vi "CANOpen_SDO List RW.vi"(8 "error in (no error)":errorcluster, 11 "SDO Asynch in":T1 {"HW Dyn Read"."Resp Chan."."Chan Refs" format="%.0x"; "HW Dyn Read"."Req Chan."."Chan Refs" format="%.0x"; "HW Dyn Write"."Resp Chan."."Chan Refs" format="%.0x"; "HW Dyn Write"."Req Chan."."Chan Refs" format="%.0x"; "List SDO"."Resp Chan."."Chan Refs" format="%.0x"; "List SDO"."Req Chan."."Chan Refs" format="%.0x"}) -> (0 "error out":errorcluster, 3 "SDO Asynch out":T1 {"HW Dyn Read"."Resp Chan."."Chan Refs" format="%.0x"; "HW Dyn Read"."Req Chan."."Chan Refs" format="%.0x"; "HW Dyn Write"."Resp Chan."."Chan Refs" format="%.0x"; "HW Dyn Write"."Req Chan."."Chan Refs" format="%.0x"; "List SDO"."Resp Chan."."Chan Refs" format="%.0x"; "List SDO"."Req Chan."."Chan Refs" format="%.0x"})   [LabVIEW 2021, in "CANOpen Addon Engine.lvlib"]
uses:
  CANOpen Addon Engine.lvlib
  CANOpen_VS SDOs Data Refs.ctl
  <vilib>/NI VeriStand/Custom Device API/Data Reference.ctl
  Async VIs/CANOpen_Main/SubVIs/CanOpen_SDO Dynamic queue.ctl
  Shared/CANOpen_SDO queue W data.ctl
  Shared/CANOpen_SDO queue mode.ctl
  Shared/CANOpen_PDO Data Type in queue.ctl
  <vilib>/NI VeriStand/Custom Device API/Global Data Refs.vi
  <vilib>/NI VeriStand/Custom Device API/Custom Device API.lvlib
  Debug/SubVIs/Global debug.vi
  <vilib>/NI VeriStand/Custom Device Tools/Custom Device Utility Library/Custom Device Utility Library.lvlib
  Shared/CANOpen Addon Shared.lvlib
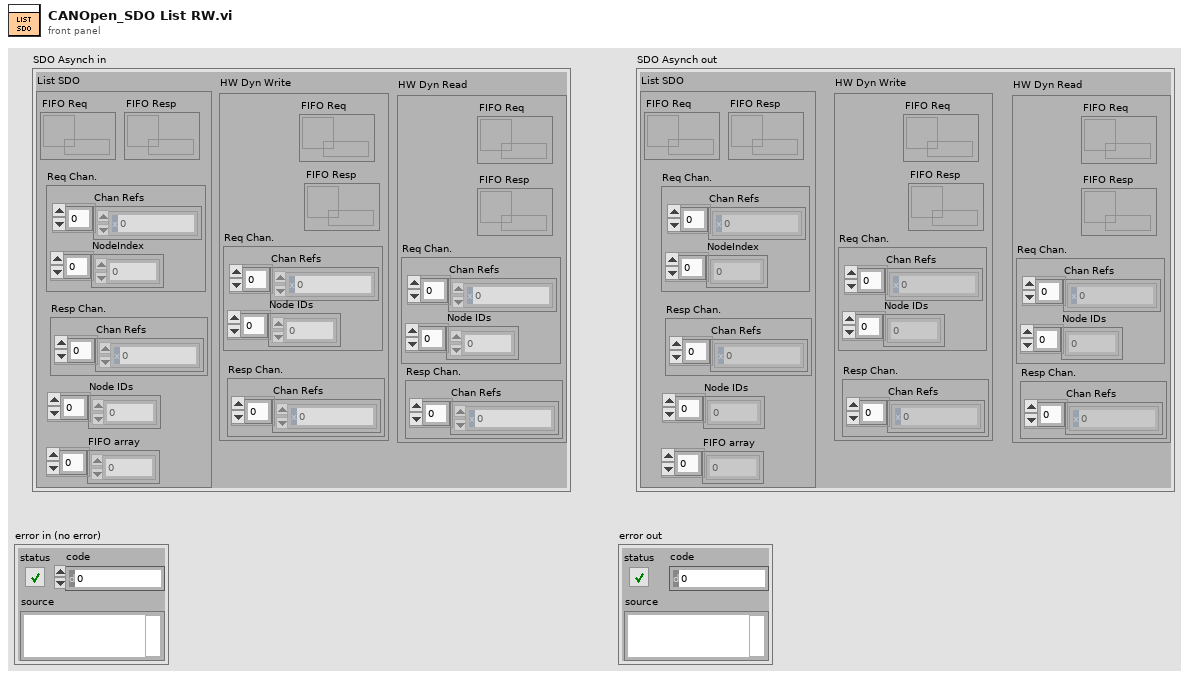
[diagram p1: front panel]
types:
  T1 = typedef "CANOpen Addon Engine.lvlib/CANOpen_VS SDOs Data Refs.ctl" = cluster{"List SDO":cluster{"FIFO Req":refnum<k33>, "Req Chan.":cluster{"Chan Refs":T2[], "NodeIndex":dbl[]}, "FIFO Resp":refnum<k33>, "Resp Chan.":cluster{"Chan Refs":T2[]}, "Node IDs":u8[], "FIFO array":dbl[]}, "HW Dyn Write":cluster{"FIFO Req":refnum<k33>, "FIFO Resp":refnum<k33>, "Req Chan.":cluster{"Chan Refs":T2[], "Node IDs":u8[]}, "Resp Chan.":cluster{"Chan Refs":T2[]}}, "HW Dyn Read":cluster{"FIFO Req":refnum<k33>, "FIFO Resp":refnum<k33>, "Req Chan.":cluster{"Chan Refs":T2[], "Node IDs":u8[]}, "Resp Chan.":cluster{"Chan Refs":T2[]}}}
  T2 = typedef "Custom Device API.lvlib/Data Reference.ctl" = i32
  T3 = typedef "CANOpen Addon Engine.lvlib/CanOpen_SDO Dynamic queue.ctl" = cluster{"Node ID":u8, "Data":T4}
  T4 = typedef "CANOpen Addon Shared.lvlib/CANOpen_SDO queue W data.ctl" = cluster{"Object Index":u16, "Object Sub-Index (0)":u8, "Mode":T5, "Data Type":T6, "Value":dbl, "Status code":dbl, "Byte Order":enum16{"big-endian, network order", "little-endian"}}
  T5 = typedef "CANOpen Addon Shared.lvlib/CANOpen_SDO queue mode.ctl" = enum16{"WRITE write", "WRITE response", "READ write", "READ response"}
  T6 = typedef "CANOpen Addon Shared.lvlib/CANOpen_PDO Data Type in queue.ctl" = enum16{"U8", "U16", "U32", "I8", "I16", "I32", "Single", "Double"}
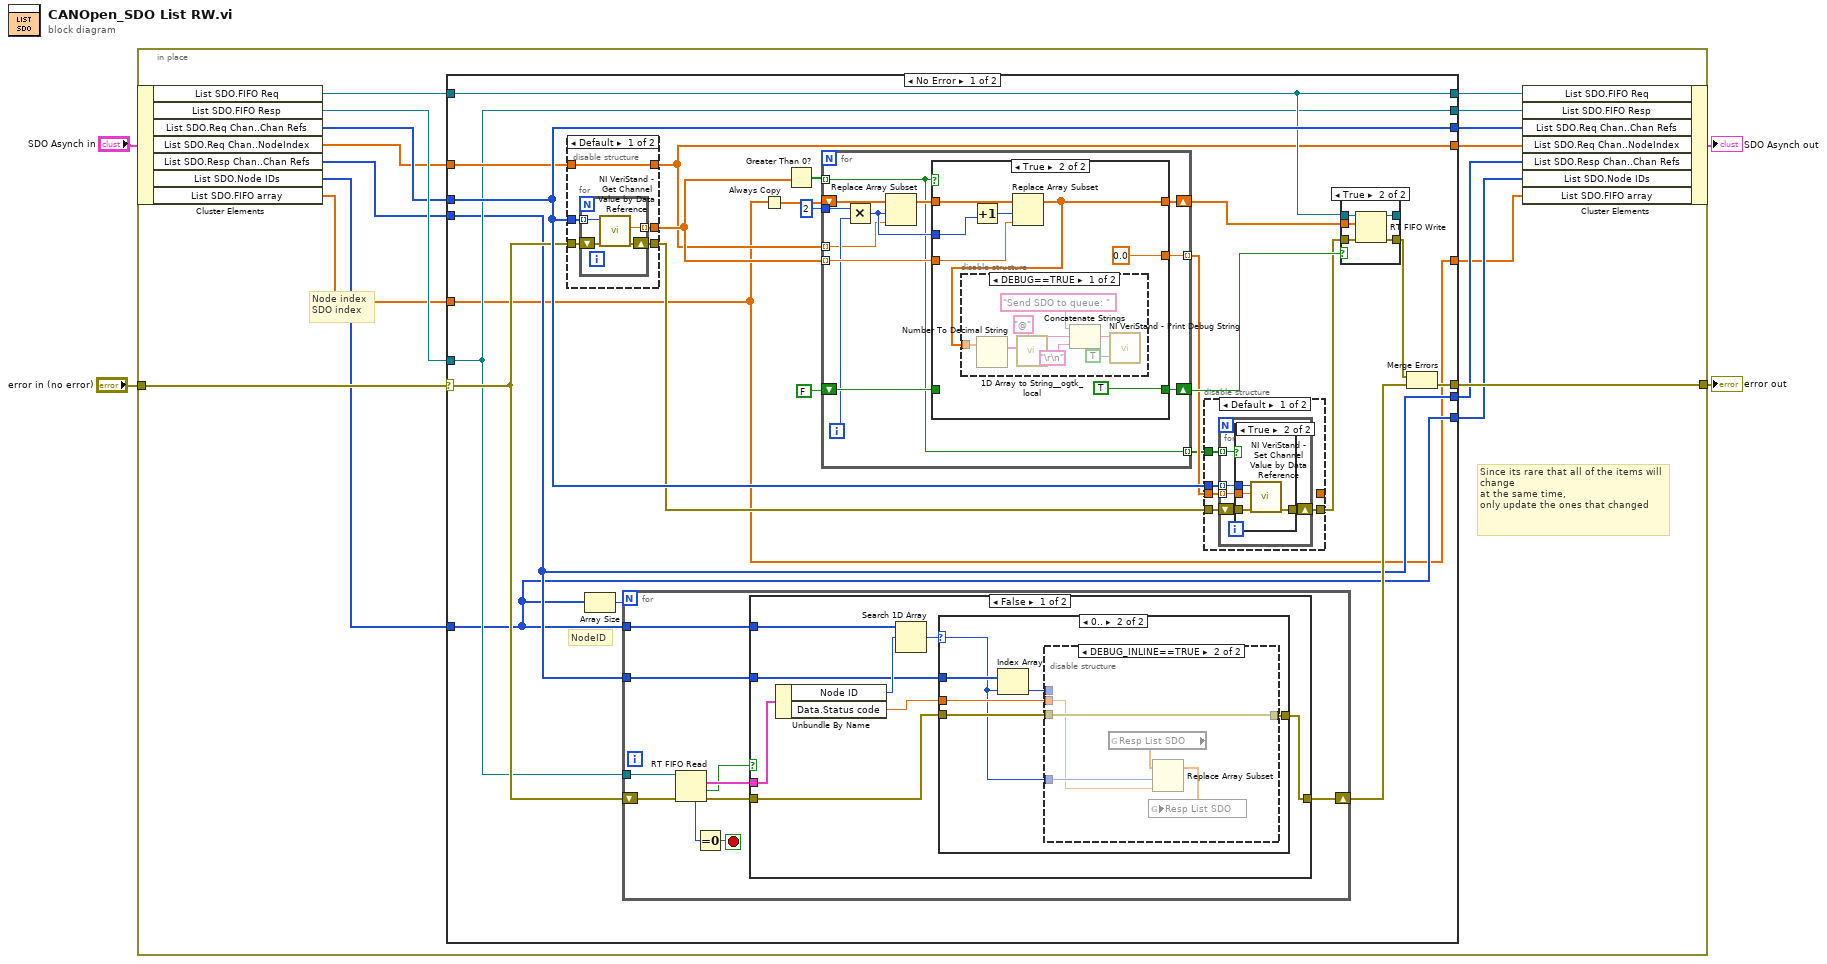
[diagram p0: block diagram]
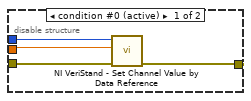
[diagram p3: hidden frame]
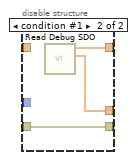
[diagram p5: hidden frame]
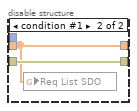
[diagram p7: hidden frame]
diagram:
  n1 = in-place {
    in-place-border: "error in (no error)" -> [w15]
    in-place-border: [w14] -> w1
    # "Since its rare that all of the items will change \nat the same time,\nonly update the ones that changed"
    # "Node index\nSDO index"
    n2 = in-place-cluster #1("SDO Asynch in") -> ("List SDO.FIFO Req"=w16:refnum<k33>, "List SDO.FIFO Resp"=w20:refnum<k33>, "List SDO.Req Chan..Chan Refs"=w18:T2[], "List SDO.Req Chan..NodeIndex"=w13:dbl[], "List SDO.Resp Chan..Chan Refs"=w9:T2[], "List SDO.Node IDs"=w7:u8[], "List SDO.FIFO array"=w6:dbl[])
    n3 = case shown="No Error" w15 {
      selector: w15 -> [w28 w149]
      tunnel: [w32 w149] -> w14
      tunnel: w20 -> [w27 w153]
      tunnel: [w27 w153] -> w19
      tunnel: w18 -> [w44 w152]
      tunnel: w13 -> [w29 w151]
      tunnel: [w44 w152] -> w17
      tunnel: [w25 w151] -> w12
      tunnel: w16 -> [w43 w150]
      tunnel: w9 -> [w26 w148]
      tunnel: [w43 w150] -> w11
      tunnel: [w26 w148] -> w10
      tunnel: w7 -> [w24 w147]
      tunnel: [w24 w147] -> w8
      tunnel: w6 -> [w21 w146]
      tunnel: [w21 w146] -> w5
      frame No Error {
        # "NodeID"
        n4 = disable-structure shown="Default" {
          disable-tunnel: w44 -> [w84 _]
          disable-tunnel: w28 -> [w83 w89]
          disable-tunnel: [w82 w89] -> w36
          disable-tunnel: [w81 w90] -> w35
          disable-tunnel: [w80 w91] -> w25
          disable-tunnel: w29 -> [w80 _]
          frame condition #0 (active) {
            n5 = for {
              tunnel: w84 -> [w88] mode=indexing
              tunnel: [w87] -> w81 mode=indexing
              shift-right: [w85] -> w82
              shift-left: w83 -> [w86]
              n6 = call <vilib>:"NI VeriStand - Get Channel Value by Data Reference.vi"("error in (no error)"=w86, "Data Reference in"=w88) -> ("error out"=w85:errorcluster, "Value"=w87:dbl)  [unwired: 8 in]
            }
          }
          frame condition #1 {
            n7 = call "Read Debug SDO.vi"() -> ("Req List SDO"=w90:dbl[], "SDO Node Index"=w91:dbl[])  [unwired: 8 in, 2 out]
          }
        }
        n8 = Array Size(array=w24) -> (size(s)=w33:i32)
        n9 = for {
          N: w33 -> [_]
          tunnel: w24 -> [w49]
          tunnel: w27 -> [w52]
          shift-right: [w46] -> w30
          shift-left: w28 -> [w51]
          tunnel: w26 -> [w48]
          stop <- w53 stop-if-true
          n10 = RT FIFO Read(0:w52, 3:w51) -> (7:w54:u32, 9:w50:T3, 10:w45:bool, 11:w47:errorcluster)  [unwired: 2 in, 1 out]
          n11 = Equal To 0?(x=w54) -> (x = 0?=w53:bool)
          n12 = case shown="False" w45 {
            tunnel: w50 -> [w62 _]
            tunnel: w49 -> [w61 _]
            tunnel: w48 -> [w58 _]
            tunnel: w47 -> [w57 w79]
            tunnel: [w56 w79] -> w46
            frame False {
              n13 = Unbundle By Name(w62) -> ("Node ID"=w60:u8, "Data.Status code"=w55:dbl)
              n14 = Search 1D Array(1D array=w61, element=w60) -> (index of element=w59:i32)  [unwired: 1 in]
              n15 = case shown="0.." w59 {
                selector: w59 -> [_ w64]
                tunnel: w58 -> [_ w69]
                tunnel: w57 -> [w63 w67]
                tunnel: [w63 w66] -> w56
                tunnel: w55 -> [_ w65]
                frame -1, Default {
                }
                frame 0.. {
                  n16 = Index Array(array=w69, index=w64) -> (element=w68:T2)
                  n17 = disable-structure shown="DEBUG_INLINE==TRUE" {
                    disable-tunnel: w68 -> [w73 _]
                    disable-tunnel: w67 -> [w72 w78]
                    disable-tunnel: [w71 w78] -> w66
                    disable-tunnel: w65 -> [w70 w76]
                    disable-tunnel: w64 -> [_ w77]
                    frame condition #0 (active) {
                      n18 = call <vilib>:"NI VeriStand - Set Channel Value by Data Reference.vi"("error in (no error)"=w72, "Value"=w70, "Data Reference in"=w73) -> ("error out"=w71:errorcluster)  [unwired: 8 in]
                    }
                    frame condition #1 {
                      n19 = global read "Global debug.vi" "Resp List SDO"() -> (w74:dbl[])
                      n20 = Replace Array Subset(array=w74, new element=w76, index=w77) -> (w75:dbl[])
                      n21 = global write "Global debug.vi" "Resp List SDO"(w75) -> ()
                    }
                  }
                }
              }
            }
            frame True {
            }
          }
        }
        n22 = Always Copy(1:w21) -> (0:w22:dbl[])
        n23 = Greater Than 0?(x=w35) -> (x > 0?=w39:bool[])
        n24 = for {
          tunnel: w39 -> [w117] mode=indexing
          tunnel: w35 -> [w127] mode=indexing
          tunnel: [w126] -> w37 mode=indexing
          shift-right: [w125] -> w41
          shift-left: FALSE -> [w124]
          tunnel: w25 -> [w116] mode=indexing
          tunnel: 2 ("x") -> [w122]
          shift-right: [w119] -> w42
          shift-left: w22 -> [w123]
          tunnel: [w117] -> w34 mode=indexing
          i -> [w121]
          n25 = Multiply(x=w122, y=w121) -> (x*y=w118:i32)
          n26 = Replace Array Subset(array=w123, new element=w116, index=w118) -> (w120:dbl[])
          n27 = case shown="True" w117 {
            tunnel: w127 -> [w130 w132]
            tunnel: [w130 0.0 ("Numeric")] -> w126
            tunnel: [w129 TRUE] -> w125
            tunnel: w124 -> [w129 _]
            tunnel: w120 -> [w128 w135]
            tunnel: [w128 w131] -> w119
            tunnel: w118 -> [_ w134]
            frame False {
            }
            frame True {
              n28 = Increment(x=w134) -> (x+1=w133:i32)
              n29 = Replace Array Subset(array=w135, new element=w132, index=w133) -> (w131:dbl[])
              n30 = disable-structure shown="DEBUG==TRUE" {
                disable-tunnel: w131 -> [w139 _]
                frame condition #0 {
                  n31 = Number To Decimal String(number=w139) -> (decimal integer string=w141:string[])  [unwired: 1 in]
                  n32 = call "1D Array to String__ogtk_local.vi"("delimiter (Tab)"="@", "Array of Strings"=w141) -> ("delimited string"=w140:string)  [unwired: 9 in]
                  n33 = Concatenate Strings("Send SDO to queue: " ("string"), w140, "\r\n") -> (w145:string)
                  n34 = call <vilib>:"NI VeriStand - Print Debug String.vi"("Add to log file? (F)"=TRUE ("Add to log file? (T)"), "Message"=w145) -> ()  [unwired: 9 in, 1 out]
                }
                frame condition #1 (active) {
                }
              }
            }
          }
        }
        n35 = disable-structure shown="Default" {
          disable-tunnel: [w96 w108] -> w38
          disable-tunnel: w36 -> [w95 w108]
          disable-tunnel: w44 -> [w94 _]
          disable-tunnel: w37 -> [w93 w107]
          disable-tunnel: [_ w107] -> _
          disable-tunnel: w34 -> [w92 _]
          frame condition #0 (active) {
            n36 = for {
              tunnel: w94 -> [w99] mode=indexing
              shift-right: [w100] -> w96
              shift-left: w95 -> [w101]
              tunnel: w93 -> [w98] mode=indexing
              tunnel: w92 -> [w97] mode=indexing
              n37 = case shown="True" w97 {
                tunnel: w101 -> [w102 w106]
                tunnel: [w102 w105] -> w100
                tunnel: w99 -> [_ w104]
                tunnel: w98 -> [_ w103]
                frame False {
                }
                frame True {
                  n38 = call <vilib>:"NI VeriStand - Set Channel Value by Data Reference.vi"("error in (no error)"=w106, "Value"=w103, "Data Reference in"=w104) -> ("error out"=w105:errorcluster)  [unwired: 8 in]
                }
              }
            }
          }
          frame condition #1 {
            n39 = global write "Global debug.vi" "Req List SDO"(w107) -> ()
          }
        }
        n40 = case shown="True" w41 {
          tunnel: [w109 w115] -> w31
          tunnel: w43 -> [w110 w114]
          tunnel: [w110 w113] -> _
          tunnel: w42 -> [_ w111]
          tunnel: w38 -> [w109 w112]
          frame False {
          }
          frame True {
            n41 = RT FIFO Write(0:w114, 1:w111, 3:w112) -> (8:w113:refnum<k33>, 11:w115:errorcluster)  [unwired: 2 in, 2 out]
          }
        }
        n42 = Merge Errors(w31, w30) -> (w32:errorcluster)
      }
      frame Error {
      }
    }
    n43 = in-place-cluster #1("List SDO.FIFO Req"=w11, "List SDO.FIFO Resp"=w19, "List SDO.Req Chan..Chan Refs"=w17, "List SDO.Req Chan..NodeIndex"=w12, "List SDO.Resp Chan..Chan Refs"=w10, "List SDO.Node IDs"=w8, "List SDO.FIFO array"=w5) -> (→"SDO Asynch out":T1)
  }
  "error out" <- w1
